vi "Init.vi"(8 "error in (no error)":errorcluster, 9 "SA Pin":string, 10 "Measurement Name":string, 11 "Standard":string) -> (0 "error out":errorcluster, 3 "Harmonics_CHP out":refnum<class "RxBN_CHP.lvclass">)   [LabVIEW 2016, in "SeqAuto Evaluations.lvlib" / "RxBN_CHP.lvclass"]
uses:
  RxBN_CHP.lvclass
  C:/projects/STS/Common/Sequence Automation/Plugins/SeqAuto IEvaluation.lvlibp/SeqAuto IEvaluation.lvclass
  RxBN_CHP.lvclass/RxBN_CHP.ctl
  Write SA Pin.vi
  Plugins/SeqAuto IEvaluation.lvlibp/Write Measurement Name.vi
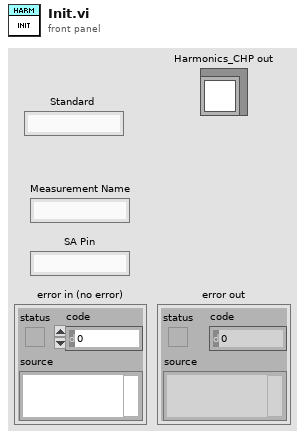
[diagram p1: front panel]
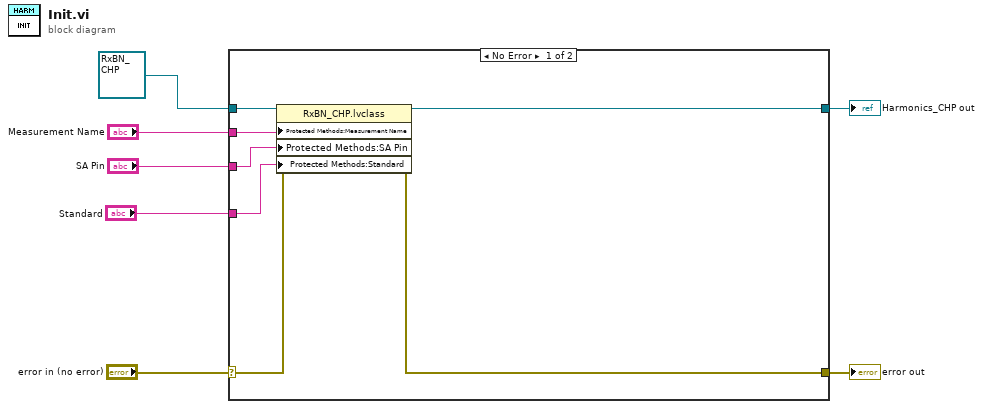
[diagram p0: block diagram]
diagram:
  n1 = case shown="No Error" "error in (no error)" {
    selector: "error in (no error)" -> [w14 w16]
    tunnel: [w13 w16] -> w6
    tunnel: [w11 w15] -> w4
    tunnel: refnum<class "RxBN_CHP.lvclass"> refnum ("Harmonics_CHP in") -> [w12 w15]
    tunnel: "Measurement Name" -> [w10 _]
    tunnel: "SA Pin" -> [w9 _]
    tunnel: "Standard" -> [w8 _]
    frame No Error {
      n2 = property class="RxBN_CHP.lvclass"(reference=w12, error in=w14, "Protected Methods:Measurement Name"=w10, "Protected Methods:SA Pin"=w9, "Protected Methods:Standard"=w8) -> (reference out=w11:refnum<class "RxBN_CHP.lvclass">, error out=w13:errorcluster)
    }
    frame Error {
    }
  }
  "error out" <- w6
  "Harmonics_CHP out" <- w4
